vi "DriveStraightTime.vi"   [LabVIEW 2016, in "DriveBase.lvclass"]
uses:
  DriveBase.lvclass
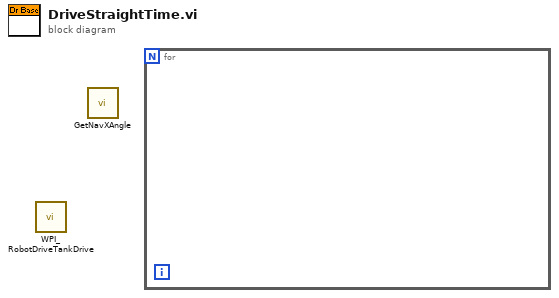
[diagram p0: block diagram]
diagram:
  n1 = call <vilib>:"WPI_RobotDriveTankDrive.vi"() -> ()  [unwired: 9 in, 3 out]
  n2 = call "GetNavXAngle.vi"() -> ()  [unwired: 10 in, 2 out]
  n3 = for {
  }
